vi "Frame rate equation.vi"(9 "Dwell time (us)":dbl, 10 "AOD fill time (us)":dbl, 11 "Frame size (single dimension)":i32) -> (3 "FrameRate (fps)":dbl)   [LabVIEW 2020]
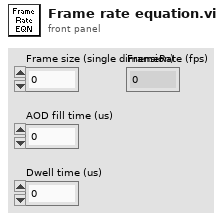
[diagram p1: front panel]
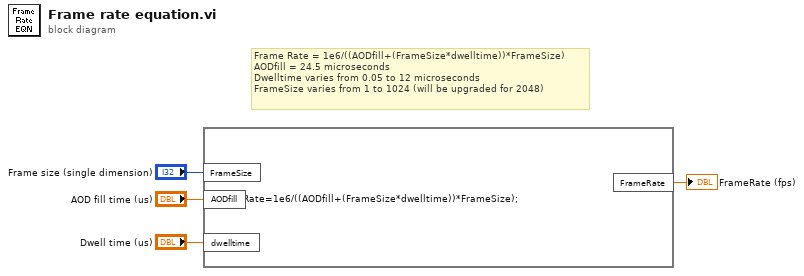
[diagram p0: block diagram]
diagram:
  # "Frame Rate = 1e6/((AODfill+(FrameSize*dwelltime))*FrameSize)\nAODfill = 24.5 microseconds \nDwelltime varies from 0.05 to 12 microseconds\nFrameSize varies from 1 to 1024 (will be upgraded for 2048)"
  n1 = formula code="FrameRate=1e6/((AODfill+(FrameSize*dwelltime))*FrameSize);"("AODfill"="AOD fill time (us)", "FrameSize"="Frame size (single dimension)", "dwelltime"="Dwell time (us)") -> ("FrameRate"=→"FrameRate (fps)":dbl)
